vi "Configure Trigger Input.vi"(6 "Trigger Slope (0: Positive)":u16(ring) items=["Positive", "Negative"], 7 "Internal Trigger Period (1 s)":dbl=1.0 min=0.005 max=100000.0, 8 "error in (no error)":errorcluster, 9 "Channel Source (0: Previous)":u16(ring) items=["Previous", "Next"], 10 "Trigger Input Source (0: Internal Trigger)":u16(ring) items=["Internal Trigger", "External Trigger", "Manual Trigger", "Channel Source"], 11 "VISA resource name":refnum<visa-resource-name>) -> (0 "error out":errorcluster, 3 "VISA resource name out":refnum<visa-resource-name>)   [LabVIEW 2015, in "Fluke 28x Series.lvlib"]
doc: "Configures settings for the various types of trigger input. These can be either internal (through another channel or through crystal oscillations), or external (through another instrument or manually).\n\n<b>Note</b>: configuring Trigger for use within the same instrument requires a multi-channel instrument, i.e. Fluke 282 or Fluke 284. Trigger can also be configured for use between generators."
uses:
  <instrlib>/Fluke 28x Series/Fluke 28x Series.lvlib
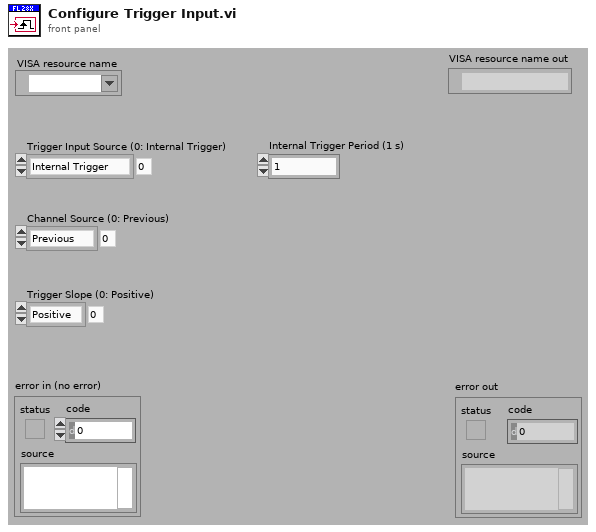
[diagram p1: front panel]
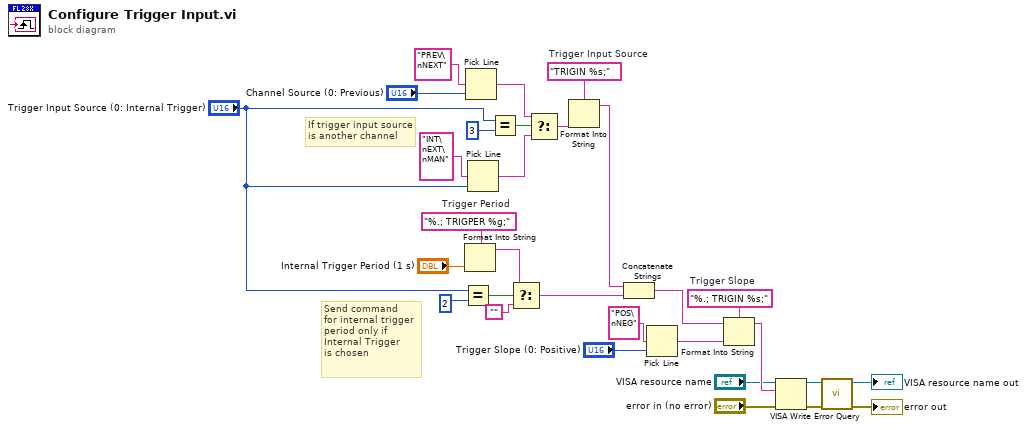
[diagram p0: block diagram]
diagram:
  w8 = "%.; TRIGPER %g;"  # Trigger Period
  w19 = "%.; TRIGIN %s;"  # Trigger Slope
  w30 = "TRIGIN %s;"  # Trigger Input Source
  # "Send command\nfor internal trigger\nperiod only if\nInternal Trigger\nis chosen"
  # "If trigger input source is another channel"
  n1 = Equal?(x="Trigger Input Source (0: Internal Trigger)", y=u16 2) -> (x = y?=w11:bool)
  n2 = Format Into String(format string=w8, "Internal Trigger Period (1 s)") -> (resulting string=w7:string)  [unwired: 2 in, 1 out]
  n3 = Pick Line(multi-line string="PREV\nNEXT", line index="Channel Source (0: Previous)") -> (output string=w26:string)  [unwired: 1 in]
  n4 = Pick Line(multi-line string="INT\nEXT\nMAN", line index="Trigger Input Source (0: Internal Trigger)") -> (output string=w24:string)  [unwired: 1 in]
  n5 = Equal?(x="Trigger Input Source (0: Internal Trigger)", y=u16 3) -> (x = y?=w14:bool)
  n6 = Select(t=w7, s=w11, f="" ("Empty String Constant")) -> (s? t:f=w5:string)
  n7 = Select(t=w26, s=w14, f=w24) -> (s? t:f=w23:string)
  n8 = Format Into String(format string=w30, w23) -> (resulting string=w6:string)  [unwired: 2 in, 1 out]
  n9 = Concatenate Strings(w6, w5) -> (w4:string)
  n10 = Pick Line(multi-line string="POS\nNEG", line index="Trigger Slope (0: Positive)") -> (output string=w20:string)  [unwired: 1 in]
  n11 = Format Into String(format string=w19, initial string=w4, w20) -> (resulting string=w18:string)  [unwired: 1 in, 1 out]
  n12 = VISA Write(VISA resource name="VISA resource name", write buffer=w18, error in (no error)="error in (no error)") -> (VISA resource name out=w15:refnum<visa-resource-name>, error out=w16:errorcluster)  [unwired: 1 out]
  n13 = call <instrlib>:"Error Query.vi"("error in (no error)"=w16, "VISA resource name"=w15) -> ("error out"=→"error out":errorcluster, "VISA resource name out"=→"VISA resource name out":refnum<visa-resource-name>)  [unwired: 6 in, 2 out]
